vi "Set Folders.vi"(8 "error in (no error)":errorcluster, 9 "Data folder":path, 10 "Calibration folder":path, 11 "State in":refnum<class "State.lvclass">) -> (0 "error out":errorcluster, 3 "State out":refnum<class "State.lvclass">)   [LabVIEW 2020, in "State.lvclass"]
uses:
  State.lvclass
  State.lvclass/State.ctl
  epl-vi-lib/Signal Synthesis VIs/4th Generation/Classes/SignalManager/SignalManager.lvclass
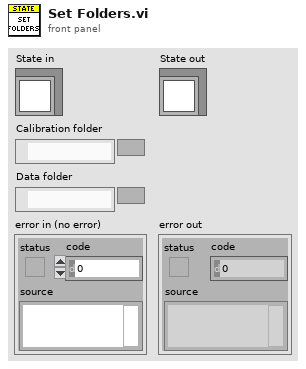
[diagram p1: front panel]
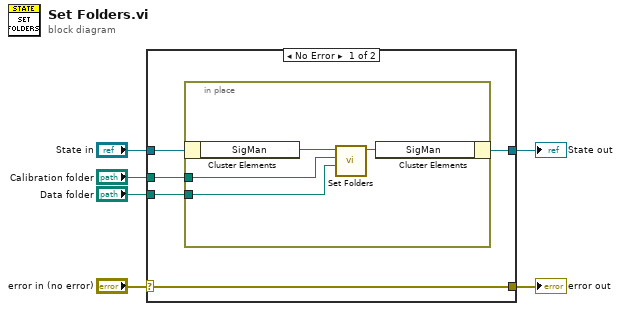
[diagram p0: block diagram]
diagram:
  n1 = case shown="No Error" "error in (no error)" {
    selector: "error in (no error)" -> [w11 w17]
    tunnel: [w11 w17] -> w5
    tunnel: [w9 w16] -> w3
    tunnel: "State in" -> [w10 w16]
    tunnel: "Calibration folder" -> [w8 _]
    tunnel: "Data folder" -> [w7 _]
    frame No Error {
      n2 = in-place {
        in-place-border: w8 -> [w13]
        in-place-border: w7 -> [w12]
        n3 = in-place-cluster #1(w10) -> ("SigMan"=w15:refnum<class "SignalManager.lvclass">)
        n4 = call "Set Folders.vi"("Local folder"=w12, "Calibration folder"=w13, "SigMan in"=w15) -> ("SigMan out"=w14:refnum<class "SignalManager.lvclass">)  [unwired: 7 in, 1 out]
        n5 = in-place-cluster #1("SigMan"=w14) -> (w9:refnum<class "State.lvclass">)
      }
    }
    frame Error {
    }
  }
  "error out" <- w5
  "State out" <- w3
